vi "Keithley 3390 Arbitrary Waveform.vi"() -> ()   [LabVIEW 2017]
doc: "This example shows how to create, configure and output an arbitrary waveform."
uses:
  Instance           1 40Saved   Keithley 3390 Arbitrary Waveform .vi
  Instance           2 40Saved   Keithley 3390 Arbitrary Waveform .vi
  Keithley 3390.lvlib
  Public/Configure/Configure Waveform (Arbitrary).vi
panel:
  in  "Offset (0.00 V)":dbl
  in  "Frequency (1000 Hz)":dbl=1000.0
  in  "Gain (1.0)":dbl=1.0
  in  "Arbitrary Waveform Name":string="ARB1"
  in  "VISA resource name":refnum<visa-resource-name>
  # "(c) 2008 Keithley Instruments, Inc.  ALL RIGHTS RESERVED."
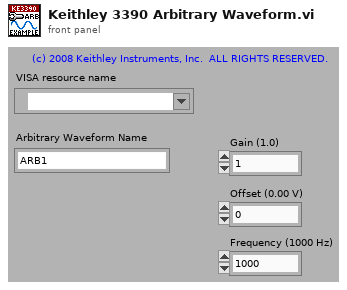
[diagram p1: front panel]
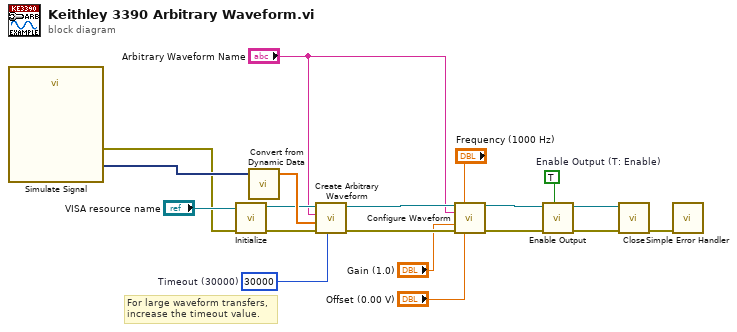
[diagram p0: block diagram]
diagram:
  w9 = TRUE  # Enable Output (T: Enable)
  w13 = u32 30000  # Timeout (30000)
  # "For large waveform transfers, increase the timeout value."
  n1 = call "Simulate Signal"() -> ("Sine"=w19:dynamicdata, "error out"=w17:errorcluster)  [unwired: 14 in]
  n2 = call "Initialize.vi"("error in (no error)"=w17, "VISA resource name"="VISA resource name") -> ("error out"=w12:errorcluster, "VISA resource name out"=w10:refnum<visa-resource-name>)  [unwired: 8 in]
  n3 = call "Convert from Dynamic Data"("Dynamic Data Type"=w19) -> ("Array"=w11:dbl[])  [unwired: 3 in]
  n4 = call "Create Arbitrary Waveform.vi"("Timeout (10000 ms)"=w13, "error in (no error)"=w12, "Arbitrary Waveform Data"=w11, "Arbitrary Waveform Name (\"ARB1\")"="Arbitrary Waveform Name", "VISA resource name"=w10) -> ("error out"=w7:errorcluster, "VISA resource name out"=w6:refnum<visa-resource-name>)  [unwired: 5 in]
  n5 = call-poly "Configure Waveform.vi"("VISA resource name"=w6, "Frequency (1000 Hz)"="Frequency (1000 Hz)", "Arbitrary Waveform Name (\"EXP_RISE\")"="Arbitrary Waveform Name", "Gain (1.0 Vpp)"="Gain (1.0)", "error in (no error)"=w7, "DC Offset (0.00 V)"="Offset (0.00 V)") -> ("VISA resource name out"=w5:refnum<visa-resource-name>, "error out"=w8:errorcluster)  [unwired: 8 in]
  n6 = call "Enable Output.vi"("Enable Output (T: Enable)"=w9, "error in (no error)"=w8, "VISA resource name"=w5) -> ("error out"=w15:errorcluster, "VISA resource name out"=w14:refnum<visa-resource-name>)  [unwired: 7 in]
  n7 = call "Close.vi"("error in (no error)"=w15, "VISA resource name"=w14) -> ("error out"=w16:errorcluster)  [unwired: 9 in]
  n8 = call <vilib>:"Simple Error Handler.vi"("error in (no error)"=w16) -> ()  [unwired: 4 in, 5 out]
